vi "Set Target.vi"(8 "error in (no error)":errorcluster, 9 "Target Rate (T/min)":dbl, 10 "Target Field (T)":dbl, 11 "Instrument.1820 in":refnum<class "Instrument.Oxford1820.lvclass">) -> (0 "error out":errorcluster, 2 "Response":string, 3 "Instrument.1820 in":refnum<class "Instrument.Oxford1820.lvclass">)   [LabVIEW 2019, in "Instrument.Oxford1820.lvclass"]
uses:
  Instrument.Oxford1820.lvclass
  Typedefs/PrivateEvents--Instrument.Oxford1820.setMagnet.ctl
  <userlib>/LevyLab/Instrument Framework/Instrument Types/Cryostat/Typedefs/Magnet Axis--Enum.ctl
  <userlib>/LevyLab/Instrument Framework/Instrument Types/Cryostat/Typedefs/Magnet Mode--Enum.ctl
  Typedefs/Instrument.Oxford1820.protectedCommands-enum.ctl
  05cfbf91-8d0b-46d2-b0f6-82182ea172bd.vi/9b5125b5-fbc3-4e2e-8507-1f471f924dba.vi
  05cfbf91-8d0b-46d2-b0f6-82182ea172bd.vi/3f3287a5-9964-4482-afeb-52cdbeb088ca.vi
  <vilib>/Utility/Data Type/Get Type Information.vi
  <vilib>/JDP Science/JSONtext/JSON text to Variant.vi
  <vilib>/JDP Science/JSONtext/LVClass Serializer/JSONtext LVClass Serializer.lvclass
  <userlib>/LevyLab/Instrument Framework/Instrument Types/Cryostat/Instrument.Cryostat.lvclass
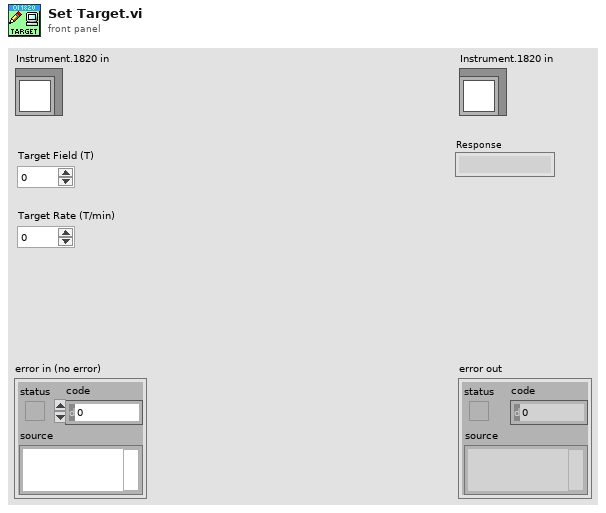
[diagram p1: front panel]
types:
  T1 = typedef "Instrument.Oxford1820.lvclass/Instrument.Oxford1820.protectedCommands-enum.ctl" = enum16{"Hold", "RampToSet", "RampToZero", "Clamp", "setTarget", "setSwitchHeat", "setLambda", "setFillMode", "setNeedleValve", "getStatus", "getTarget", "getSwitchHeat", "getPSUField", "setSequenceStatus"}
  T2 = typedef "Instrument.Oxford1820.lvclass/PrivateEvents--Instrument.Oxford1820.setMagnet.ctl" = cluster{"field":dbl, "rate":dbl, "axis":T3, "mode":T4}
  T3 = typedef "Instrument.Cryostat.lvclass/Magnet Axis--Enum.ctl" = enum16{"X", "Y", "Z"}
  T4 = typedef "Instrument.Cryostat.lvclass/Magnet Mode--Enum.ctl" = enum16{"Persistent", "Driven"}
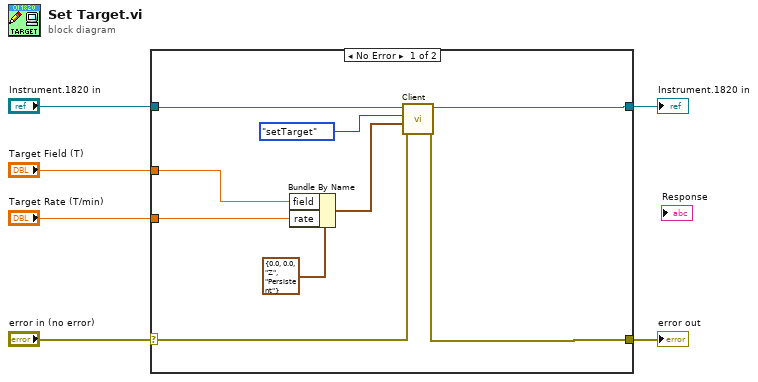
[diagram p0: block diagram]
diagram:
  n1 = case shown="No Error" "error in (no error)" {
    selector: "error in (no error)" -> [w9 w17]
    tunnel: "Target Rate (T/min)" -> [w15 _]
    tunnel: [w7 w17] -> w5
    tunnel: "Target Field (T)" -> [w14 _]
    tunnel: "Instrument.1820 in" -> [w11 w16]
    tunnel: [w10 w16] -> w1
    frame No Error {
      n2 = Bundle By Name(cluster=T2 {"field"=0.0, "rate"=0.0, "axis"=enum."Z", "mode"=enum."Persistent"} ("Set Magnet Field"), "field"=w14, "rate"=w15) -> (w12:T2)
      n3 = call-dynamic "Client.vi"("error in (no error)"=w9, "Data in"=w12, "Command in"=Instrument.Oxford1820.protectedCommands-enum."setTarget" ("Commands"), "Instrument in"=w11) -> ("error out"=w7:errorcluster, "Instrument out"=w10:refnum<class "Instrument.Oxford1820.lvclass">)  [unwired: 4 in, 2 out]
    }
    frame Error {
    }
  }
  "Instrument.1820 in" <- w1
  "error out" <- w5
